vi "Attributes name to terminal name.vi"(2 "Attributes Name":T1) -> (0 "terminal Name":string, 1 "Terminal ID":string)   [LabVIEW 2020, in "GetSetShared.lvlib"]
uses:
  <vilib>/express/express signal manip/GetorSetDDTAttributes/Shared VIs/GetSetShared.lvlib
  <vilib>/express/express signal manip/GetorSetDDTAttributes/Shared VIs/Attributes name.ctl
  <vilib>/express/express signal manip/GetorSetDDTAttributes/Shared VIs/Global 1.vi
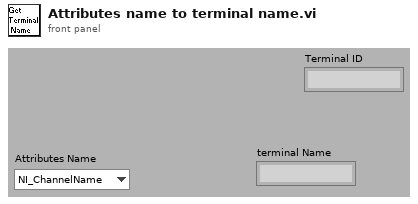
[diagram p1: front panel]
types:
  T1 = typedef "GetSetShared.lvlib/Attributes name.ctl" = enum16{"NI_ChannelName", "NI_ExpIsRelativeTime", "NI_ExpTimeStamp", "NI_ExpStartTimeStamp", "NI_ExpXDimension", "NI_UnitDescription"}
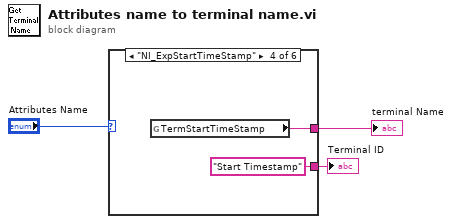
[diagram p0: block diagram]
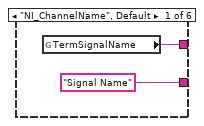
[diagram p2: hidden frame]
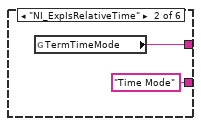
[diagram p3: hidden frame]
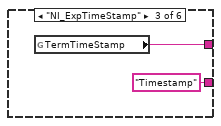
[diagram p4: hidden frame]
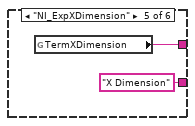
[diagram p5: hidden frame]
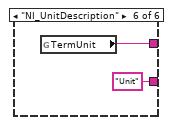
[diagram p6: hidden frame]
diagram:
  n1 = case shown="\"NI_ExpStartTimeStamp\"" "Attributes Name" {
    tunnel: [w5 w7 w9 w11 w13 w15] -> w2
    tunnel: ["Signal Name" "Time Mode" "Timestamp" "Start Timestamp" "X Dimension" "Unit"] -> w1
    frame "NI_ChannelName", Default {
      n2 = global read "Global 1.vi" "TermSignalName"() -> (w5:string)
    }
    frame "NI_ExpIsRelativeTime" {
      n3 = global read "Global 1.vi" "TermTimeMode"() -> (w7:string)
    }
    frame "NI_ExpTimeStamp" {
      n4 = global read "Global 1.vi" "TermTimeStamp"() -> (w9:string)
    }
    frame "NI_ExpStartTimeStamp" {
      n5 = global read "Global 1.vi" "TermStartTimeStamp"() -> (w11:string)
    }
    frame "NI_ExpXDimension" {
      n6 = global read "Global 1.vi" "TermXDimension"() -> (w13:string)
    }
    frame "NI_UnitDescription" {
      n7 = global read "Global 1.vi" "TermUnit"() -> (w15:string)
    }
  }
  "terminal Name" <- w2
  "Terminal ID" <- w1
